vi "rqcAlice Pseudo SPI (FPGA).vi"(0 "data in":u32, 9 "write":bool) -> (4 "data":bool, 6 "we":bool, 8 "clk":bool)   [LabVIEW 2018]
uses:
  Custom Controls/Pseudo SPI/rqcAlice PS state cluster.ctl
  Custom Controls/Pseudo SPI/rqcAlice PS states.ctl
panel:
  in  "voa":bool
  in  "MSB first":bool=TRUE
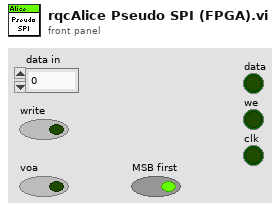
[diagram p1: front panel]
types:
  T1 = typedef "rqcAlice PS state cluster.ctl" = cluster{"data":bool[], "state":T2, "spi.data":bool, "spi.we":bool, "spi.clk":bool, "bits sent":u8}
  T2 = typedef "rqcAlice PS states.ctl" = enum16{"idle", "send"}
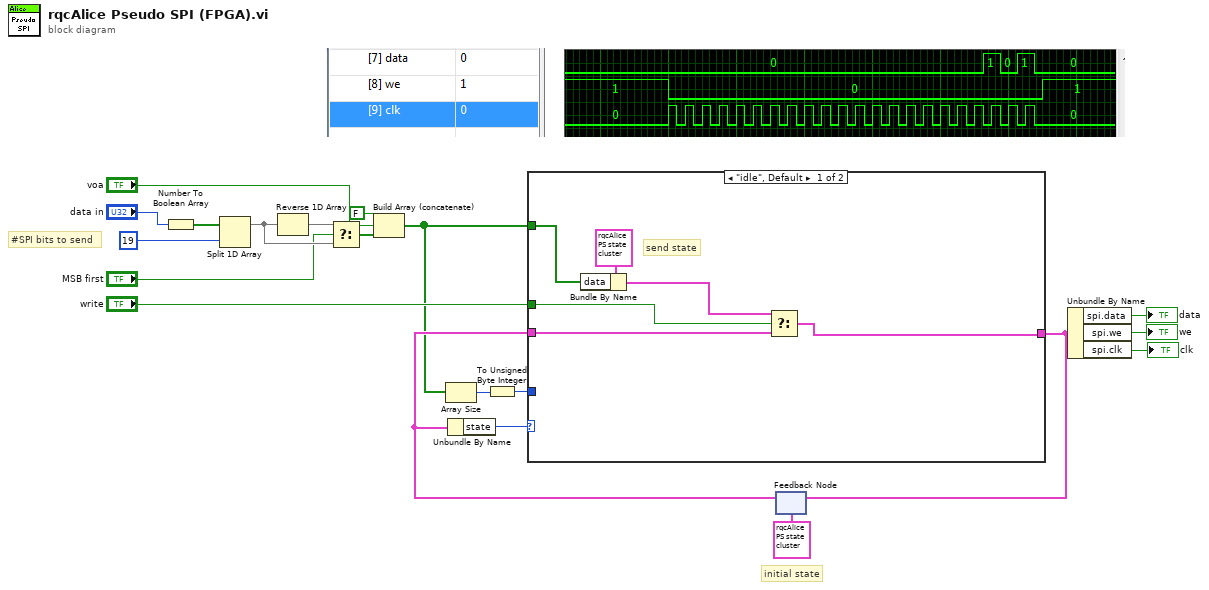
[diagram p0: block diagram]
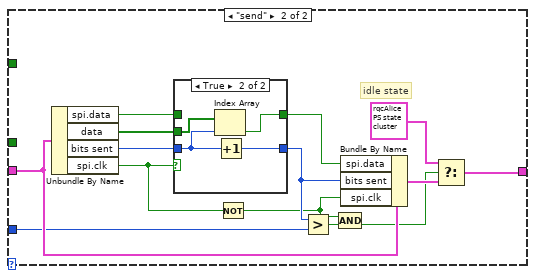
[diagram p2: hidden frame]
diagram:
  # "initial state"
  # "#SPI bits to send"
  n1 = Number To Boolean Array(number="data in") -> (Boolean array=w19:bool[])
  n2 = Split 1D Array(array=w19, index=u8 19) -> (first subarray=w18:bool[])  [unwired: 1 out]
  n3 = Reverse 1D Array(array=w18) -> (reversed array=w6:bool[])
  n4 = Select(t=w6, s="MSB first", f=w18) -> (s? t:f=w15:bool[])
  n5 = Build Array (concatenate)(FALSE ("element"), "voa", w15) -> (w3:bool[])
  n6 = Array Size(array=w3) -> (size(s)=w4:i32)
  n7 = To Unsigned Byte Integer(number=w4) -> (unsigned 8bit integer=w2:u8)
  n8 = feedback #1(T1 {"data"=[FALSE, FALSE, FALSE, FALSE, FALSE, FALSE, FALSE, FALSE, FALSE, FALSE, FALSE, FALSE, FALSE, FALSE, FALSE, FALSE, FALSE, FALSE, FALSE, FALSE, FALSE], "state"=enum."idle", "spi.data"=FALSE, "spi.we"=TRUE, "spi.clk"=FALSE, "bits sent"=0} ("PS state cluster")) -> (w12:T1)
  n9 = Unbundle By Name(w12) -> ("state"=w13:T2)
  n10 = case shown="\"idle\", Default" w13 {
    tunnel: w2 -> [_ w34]
    tunnel: w3 -> [w24 _]
    tunnel: "write" -> [w23 _]
    tunnel: [w22 w31] -> w11
    tunnel: w12 -> [w21 w40]
    frame "idle", Default {
      # "send state"
      n11 = Bundle By Name(cluster=T1 {"data"=[FALSE, FALSE, FALSE, FALSE, FALSE, FALSE, FALSE, FALSE, FALSE, FALSE, FALSE, FALSE, FALSE, FALSE, FALSE, FALSE, FALSE, FALSE, FALSE, FALSE, FALSE], "state"=enum."send", "spi.data"=FALSE, "spi.we"=FALSE, "spi.clk"=TRUE, "bits sent"=0} ("PS state cluster"), "data"=w24) -> (w26:T1)
      n12 = Select(t=w26, s=w23, f=w21) -> (s? t:f=w22:T1)
    }
    frame "send" {
      # "idle state"
      n13 = Unbundle By Name(w40) -> ("spi.data"=w37:bool, "data"=w39:bool[], "bits sent"=w38:u8, "spi.clk"=w33:bool)
      n14 = case shown="True" w33 {
        tunnel: w39 -> [_ w46]
        tunnel: w38 -> [w41 w44]
        tunnel: [w42 w45] -> w36
        tunnel: w37 -> [w42 _]
        tunnel: [w41 w43] -> w35
        frame False {
        }
        frame True {
          n15 = Index Array(array=w46, index=w44) -> (element=w45:bool)
          n16 = Increment(x=w44) -> (x+1=w43:u8)
        }
      }
      n17 = Not(x=w33) -> (.not. x?=w27:bool)
      n18 = Greater?(x=w35, y=w34) -> (0:w32:bool)
      n19 = Compound Arithmetic op=AND(w27, w32) -> (w28:bool)
      n20 = Bundle By Name(cluster=w40, "spi.data"=w36, "bits sent"=w35, "spi.clk"=w27) -> (w30:T1)
      n21 = Select(t=T1 {"data"=[FALSE, FALSE, FALSE, FALSE, FALSE, FALSE, FALSE, FALSE, FALSE, FALSE, FALSE, FALSE, FALSE, FALSE, FALSE, FALSE, FALSE, FALSE, FALSE, FALSE, FALSE], "state"=enum."idle", "spi.data"=FALSE, "spi.we"=TRUE, "spi.clk"=FALSE, "bits sent"=0} ("PS state cluster"), s=w28, f=w30) -> (s? t:f=w31:T1)
    }
  }
  n22 = feedback-in #1(w11) -> ()
  n23 = Unbundle By Name(w11) -> ("spi.data"=→"data":bool, "spi.we"=→"we":bool, "spi.clk"=→"clk":bool)
